vi "Agilent 3458 Acquire Multiple(Math) Measurement.vi"() -> ()   [LabVIEW 2010]
doc: "Shows how to configure and take multiple measurements with the math scale function applied to each measurement."
uses:
  <instrlib>/Agilent 3458/Public/Data/Read Measurement(Multiple Points).vi
  <instrlib>/Agilent 3458/Agilent 3458.lvlib
panel:
  in  "Manual Range (1.00)":dbl=1.0 format="%_3g"
  in  "Trigger Count (1)":dbl=1.0
  in  "Sample Count (1)":dbl=10.0 format="%#.6g"
  out "Measurements":sgl[](array[numeric])
  in  "Scale Value (1.00)":dbl=1.0 format="%_3g"
  in  "Trigger Type (0:Auto)":u16(ring) items=["Auto", "External", "Level", "Line", "Synchronous"]
  in  "Auto Range (1:ON)":u16(ring)=1 items=["OFF", "ON", "ONCE"]
  in  "Manual Resolution (2: 6.5 digits)":enum16{"4.5", "5.5", "6.5", "7.5", "8.5"}(ring)=enum."6.5"
  in  "Frequency Source (3: ACV)":u16(ring)=3 items=["ACDCI", "ACDCV", "ACI", "ACV"]
  in  "Maximum Time (10000 ms)":u32=10000
  in  "Function (0: DC Voltage)":u16(ring) items=["DC Voltage", "AC Voltage", "AC + DC Voltage", "DC Current", "AC Current", "AC + DC Current", "2-Wire Resistance", "4-Wire Resistance", "Frequency", "Period", "Direct Sampling DC", "Direct Sampling AC"]
  in  "VISA resource name":refnum<visa-resource-name>
  # "(c) 2007  National Instruments.  ALL RIGHTS RESERVED."
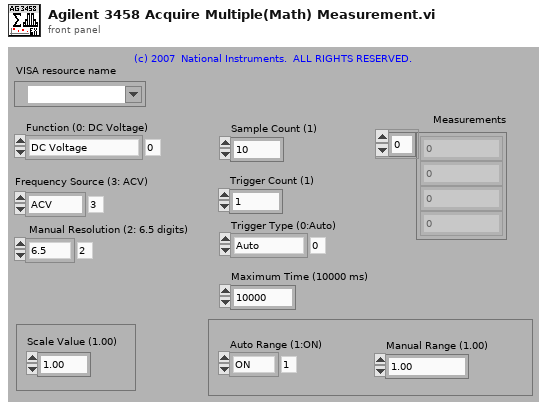
[diagram p1: front panel]
types:
  T1 = enum16{"CRTD85", "CRTD92", "CTHRM", "CTHRM2K", "CTHRM10K", "dB", "dBm", "Filter", "FRTD85", "FRTD92", "FTHRM", "FTHRM2K", "FTHRM10K", "None", "Null", "Pass/Fail", "Percent", "RMS", "Scale", "Statistics"}
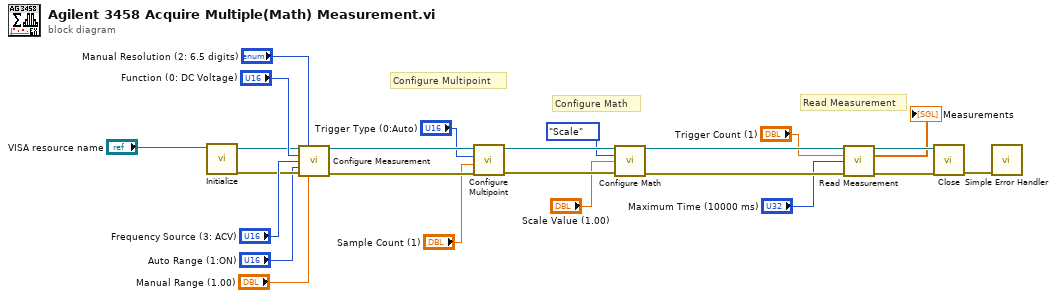
[diagram p0: block diagram]
diagram:
  # "Configure Multipoint"
  # "Read Measurement"
  # "Configure Math"
  n1 = call <instrlib>:"Initialize.vi"("VISA resource name"="VISA resource name") -> ("error out"=w12:errorcluster, "VISA resource name out"=w13:refnum<visa-resource-name>)  [unwired: 9 in]
  n2 = call <instrlib>:"Configure Measurement.vi"("VISA resource name"=w13, "Manual Resolution (2: 6.5 digits)"="Manual Resolution (2: 6.5 digits)", "Function (0: DC Voltage)"="Function (0: DC Voltage)", "Frequency Source (3: AC Voltage)"="Frequency Source (3: ACV)", "Auto Range (1:ON)"="Auto Range (1:ON)", "error in (no error)"=w12, "Manual Range (1.00)"="Manual Range (1.00)") -> ("VISA resource name out"=w17:refnum<visa-resource-name>, "error out"=w16:errorcluster)  [unwired: 7 in]
  n3 = call <instrlib>:"Configure Multipoint.vi"("error in (no error)"=w16, "Sample Count (1)"="Sample Count (1)", "Trigger Type (0:Auto)"="Trigger Type (0:Auto)", "VISA resource name"=w17) -> ("error out"=w14:errorcluster, "VISA resource name out"=w15:refnum<visa-resource-name>)  [unwired: 6 in]
  n4 = call <instrlib>:"Configure Math.vi"("VISA resource name"=w15, "Operation (13:None)"=T1."Scale", "Scale Value (1.00)"="Scale Value (1.00)", "error in (no error)"=w14) -> ("VISA resource name out"=w24:refnum<visa-resource-name>, "error out"=w23:errorcluster)  [unwired: 10 in]
  n5 = call-poly <instrlib>:"Read Measurement.vi"("VISA resource name"=w24, "Trigger Count (1)"="Trigger Count (1)", "Maximum Time (10000 ms)"="Maximum Time (10000 ms)", "error in (no error)"=w23) -> ("VISA resource name out"=w11:refnum<visa-resource-name>, "Measurements"=→"Measurements":sgl[], "error out"=w10:errorcluster)  [unwired: 9 in]
  n6 = call <instrlib>:"Close.vi"("error in (no error)"=w10, "VISA resource name"=w11) -> ("error out"=w22:errorcluster)  [unwired: 9 in]
  n7 = call <vilib>:"Simple Error Handler.vi"("error in (no error)"=w22) -> ()  [unwired: 4 in, 5 out]
